vi "Close.vi"(8 "error in (no error)":errorcluster, 11 "FTP in":refnum<class "FTP.lvclass">) -> (0 "error out":errorcluster)   [LabVIEW 2015, in "RT Management.lvlib" / "FTP.lvclass"]
uses:
  FTP.lvclass
  FTP.lvclass/FTP.ctl
  Get Session.vi
  <vilib>/FTP/NI_FTP.lvlib
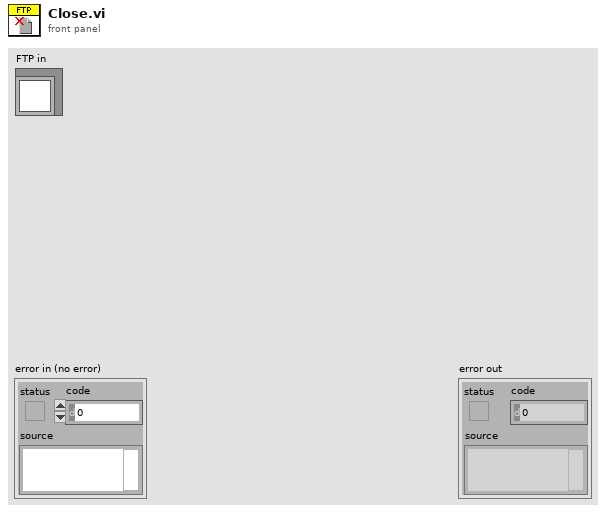
[diagram p1: front panel]
types:
  T1 = typedef "NI_FTP.lvlib/FTP Session.ctl" = refnum<k5>
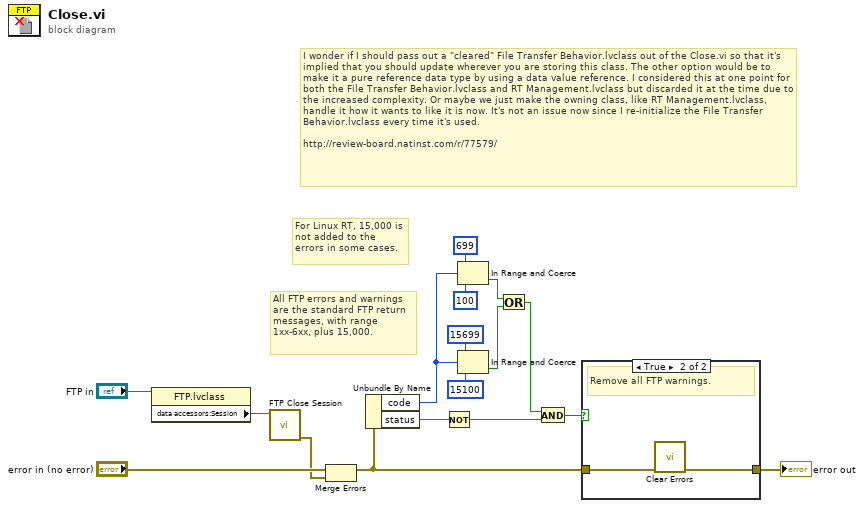
[diagram p0: block diagram]
diagram:
  # "I wonder if I should pass out a \"cleared\" File Transfer Behavior.lvclass out of the Close.vi so that it's implied that you should update wherever you are storing this class. The other option would be to make it a pure reference data type by using a data value reference. I considered this at one point for both the File Transfer Behavior.lvclass and RT Management.lvclass but discarded it at the time due to the increased complexity. Or maybe we just make the owning class, like RT Management.lvclass, handle it how it wants to like it is now. It's not an issue now since I re-initialize the File Transfer Behavior.lvclass every time it's used.\n\nhttp://review-board.natinst.com/r/77579/"
  # "For Linux RT, 15,000 is not added to the errors in some cases."
  # "All FTP errors and warnings are the standard FTP return messages, with range 1xx-6xx, plus 15,000."
  n1 = property class="FTP.lvclass"(reference="FTP in") -> ("data accessors:Session"=w16:T1)  [unwired: 1 in, 2 out]
  n2 = call <vilib>:"FTP Close Session.vi"("ftp session"=w16) -> ("error out"=w14:errorcluster)  [unwired: 7 in, 3 out]
  n3 = Merge Errors("error in (no error)", w14) -> (w1:errorcluster)
  n4 = Unbundle By Name(w1) -> ("code"=w6:i32, "status"=w13:bool)
  n5 = Not(x=w13) -> (.not. x?=w9:bool)
  n6 = In Range and Coerce(upper limit=699, x=w6, lower limit=100) -> (In Range?=w5:bool)  [unwired: 1 out]
  n7 = In Range and Coerce(upper limit=15699, x=w6, lower limit=15100) -> (In Range?=w4:bool)  [unwired: 1 out]
  n8 = Or(x=w5, y=w4) -> (x .or. y?=w3:bool)
  n9 = And(x=w3, y=w9) -> (x .and. y?=w2:bool)
  n10 = case shown="True" w2 {
    tunnel: [w18 w20] -> w12
    tunnel: w1 -> [w18 w19]
    frame False {
    }
    frame True {
      # "Remove all FTP warnings."
      n11 = call <vilib>:"Clear Errors.vi"("error in (no error)"=w19) -> ("error out"=w20:errorcluster)  [unwired: 5 in, 1 out]
    }
  }
  "error out" <- w12
